vi "Create One Timeset.vi"(6 "timeset name":string="-", 7 "Notes":string, 8 "error in (no error)":errorcluster, 9 "Pin State":T1[](array[typedef]), 10 "opcode":string, 11 "BML_LS Pattern Creator in":refnum<class "BML_LS Pattern Creator.lvclass">) -> (0 "error out":errorcluster, 2 "string out":string, 3 "BML_LS Pattern Creator out":refnum<class "BML_LS Pattern Creator.lvclass">)   [LabVIEW 2018, in "BML_LS Pattern Creator.lvlib" / "BML_LS Pattern Creator.lvclass"]
uses:
  BML_LS Pattern Creator.lvclass
  Interfaces/Protocol Interface.lvlibp/Interfaces/Protocol Interface/Pin State.ctl
  Interfaces/Protocol Interface.lvlibp/Interfaces/Protocol Interface/Protocol Interface.lvclass
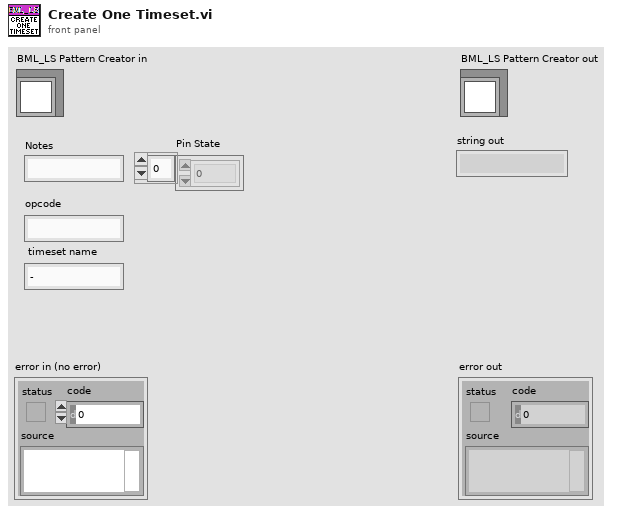
[diagram p1: front panel]
types:
  T1 = typedef "Protocol Interface.lvlibp/Protocol Interface.lvclass/Pin State.ctl" = enum16{"0", "1", "L", "H", "X", "V", "D", "M"}
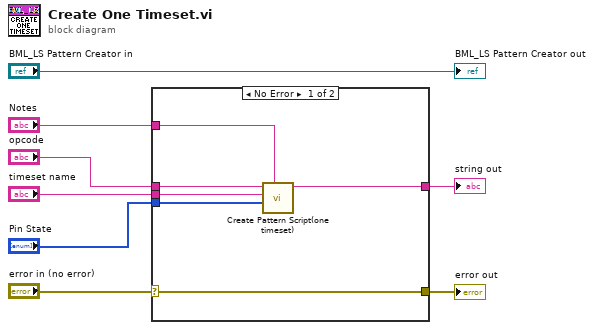
[diagram p0: block diagram]
diagram:
  n1 = case shown="No Error" "error in (no error)" {
    selector: "error in (no error)" -> [w9 w15]
    tunnel: [w9 w15] -> w7
    tunnel: "Pin State" -> [w14 _]
    tunnel: "timeset name" -> [w13 _]
    tunnel: "opcode" -> [w12 _]
    tunnel: "Notes" -> [w11 _]
    tunnel: [w10 _] -> w1
    frame No Error {
      n2 = call "Create Pattern Script(one timeset).vi"("Notes"=w11, "Pin States"=w14, "timeset name"=w13, "opcode"=w12) -> ("string out"=w10:string)  [unwired: 7 in]
    }
    frame Error {
    }
  }
  "error out" <- w7
  "string out" <- w1
  "BML_LS Pattern Creator out" <- "BML_LS Pattern Creator in"
